vi "Solartron 1260 freq scan.vi"(0 "VISA resource name":refnum<visa-resource-name>, 11 "error in (no error)":errorcluster) -> ()   [LabVIEW 2014]
doc: "This VI configures and reads back a single measurement. \n\nNote:\nYou might need to extend the timeout set in the Wait Conditions subVI."
uses:
  <vilib>/Utility/file.llb/Write To Spreadsheet File (string).vi
  <instrlib>/Solartron 1260/Solartron 1260.lvlib
panel:
  out "scan time (hrs)":dbl
  out "scan time (min)":dbl
  in  "stop":bool
  out "resonant freq (Hz)":dbl format="%#_13f"
  out "Step size (Hz)":dbl
  out "XY Graph 3":cluster{dbl[], dbl[]}[](graph)
  in  "Frequency options":T1 {"Start freq (Hz)" format="%#_8f"; "End freq (Hz)" format="%#_8f"}
  in  "Cluster":cluster{"DC Bias (V)":dbl, "Amplitude (V)":dbl}={"DC Bias (V)"=0.0, "Amplitude (V)"=1.0} {"Amplitude (V)" min=0.0 max=3.0 format="%^.3e"; "DC Bias (V)" min=-42.0 max=42.0 format="%^.3e"}
  in  "Variable, result source, citcuit":T2
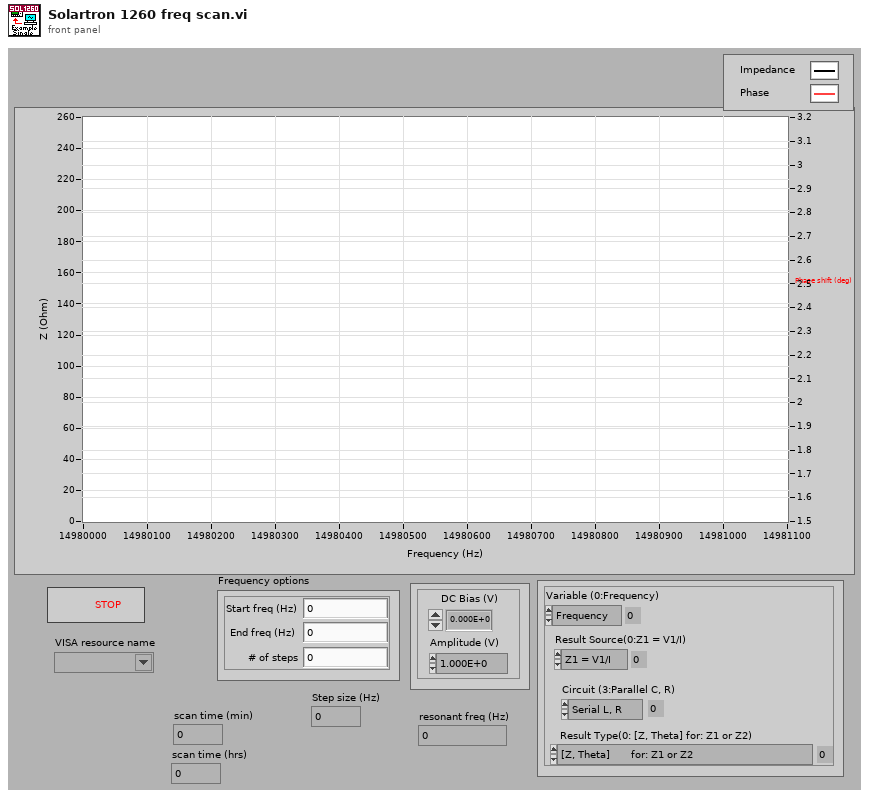
[diagram p1: front panel]
types:
  T1 = cluster{"End freq (Hz)":dbl, "Start freq (Hz)":dbl, "# of steps":dbl}
  T2 = cluster{"Variable (0:Frequency)":enum16{"Frequency", "Amplitude", "Baise"}, "Result Source(0:Z1 = V1/I)":enum16{"Z1 = V1/I", "Y1 = I/V1", "Z2 = V2/I", "Y2 = I/V2", "Function (  )", "V1", "V2", "V1/V2", "V2/V1", " I"}, "Circuit (3:Parallel C, R)":enum16{"Serial L, R", "Serial C, R", "Parallel L, R", "Parallel C, R", "Auto"}, "Result Type(0: [Z, Theta] for: Z1 or Z2)":enum16{"[Z, Theta]       for: Z1 or Z2", "[Y, Theta]       for: Y1 or Y2", "[r, Theta]        for: Fnc( ), V1, V2, V1/V2, V2/V1 or I", "[r(dB), Theta]  for: Fnc( ), V1, V2, V1/V2 or V2/V1", "[r, t]                 for: Fnc( ), V1, V2, V1/V2 or V2/V1", "[r (dB), t]          for: Fnc( ), V1, V2, V1/V2 or V2/V1", "[L(or C), R]      for: Z1, Y1, Z2, Y2 or Fnc( )", "[L(or C), Q]      for: Z1, Y1, Z2, Y2 or Fnc( )", "[L(or C), D]      for: Z1, Y1, Z2, Y2 or Fnc( ) ", "[R, X]              for: Z1 or Z2", "[G, B]              for: Y1 or Y2", "[a, b]               for: Fnc( ), V1, V2, V1/V2, V2/V1 or I"}}
  T3 = enum16{"Off", "All", "Fail", "Pass", "Dump", "Dump all", "Plotter"}
  T4 = enum16{"Z1 = V1/I", "Y1 = I/V1", "Z2 = V2/I", "Y2 = I/V2", "Function (  )", "V1", "V2", "V1/V2", "V2/V1", " I"}
  T5 = enum16{"Serial L, R", "Serial C, R", "Parallel L, R", "Parallel C, R", "Auto"}
  T6 = enum16{"[Z, Theta]       for: Z1 or Z2", "[Y, Theta]       for: Y1 or Y2", "[r, Theta]        for: Fnc( ), V1, V2, V1/V2, V2/V1 or I", "[r(dB), Theta]  for: Fnc( ), V1, V2, V1/V2 or V2/V1", "[r, t]                 for: Fnc( ), V1, V2, V1/V2 or V2/V1", "[r (dB), t]          for: Fnc( ), V1, V2, V1/V2 or V2/V1", "[L(or C), R]      for: Z1, Y1, Z2, Y2 or Fnc( )", "[L(or C), Q]      for: Z1, Y1, Z2, Y2 or Fnc( )", "[L(or C), D]      for: Z1, Y1, Z2, Y2 or Fnc( ) ", "[R, X]              for: Z1 or Z2", "[G, B]              for: Y1 or Y2", "[a, b]               for: Fnc( ), V1, V2, V1/V2, V2/V1 or I"}
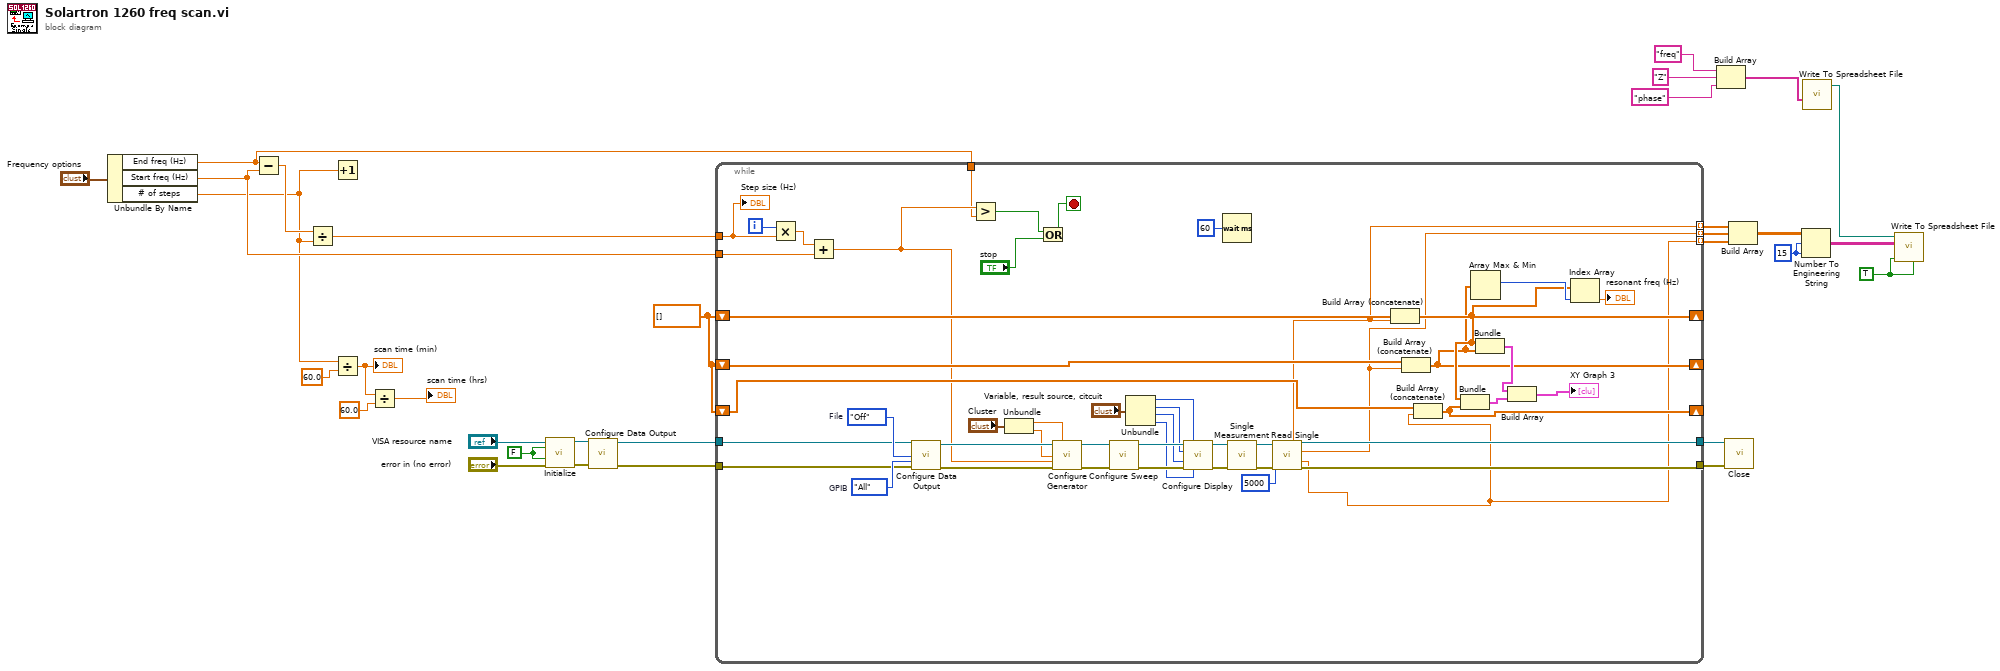
[diagram p0: block diagram]
diagram:
  w6 = TRUE ("append to file? (new file:F)")
  w14 = i16 15 ("precision (6)")
  w19 = dbl[] []
  w29 = FALSE ("ID Query (T: Check)")
  n1 = Unbundle By Name("Frequency options") -> ("End freq (Hz)"=w7:dbl, "Start freq (Hz)"=w21:dbl, "# of steps"=w4:dbl)
  n2 = Subtract(x=w7, y=w21) -> (x-y=w32:dbl)
  n3 = Divide(x=w32, y=w4) -> (x/y=w20:dbl)
  n4 = Increment(x=w4) -> ()  [unwired: 1 out]
  n5 = Divide(x=w4, y=60.0) -> (x/y=w2:dbl)
  "scan time (min)" <- w2
  n6 = Divide(x=w2, y=60.0) -> (x/y=→"scan time (hrs)":dbl)
  n7 = call <instrlib>:"Initialize.vi"("VISA resource name"="VISA resource name", "ID Query (T: Check)"=w29, "Reset (T: Reset)"=w29, "error in (no error)"="error in (no error)") -> ("VISA resource name out"=w25:refnum<visa-resource-name>, "error out"=w26:errorcluster)  [unwired: 10 in]
  n8 = call <instrlib>:"Configure Data Output.vi"("VISA resource name"=w25, "error in (no error)"=w26) -> ("VISA resource name out"=w24:refnum<visa-resource-name>, "error out"=w23:errorcluster)  [unwired: 12 in]
  n9 = while {
    tunnel: [w62] -> w31
    tunnel: [w61] -> w30
    tunnel: w24 -> [w64]
    tunnel: w23 -> [w63]
    tunnel: w21 -> [w78]
    shift-right: [w43] -> _
    shift-left: w19 -> [w60]
    shift-right: [w41] -> _
    shift-left: w19 -> [w59]
    tunnel: w20 -> [w50]
    shift-right: [w46] -> _
    shift-left: w19 -> [w47]
    tunnel: [w40] -> w18 mode=indexing
    tunnel: [w34] -> w17 mode=indexing
    tunnel: [w33] -> w16 mode=indexing
    tunnel: w7 -> [w36]
    i -> [w80]
    stop <- w39 stop-if-true
    w66 = T3."All"  # GPIB
    w67 = enum16{"Off", "All", "Fail", "Pass"}."Off"  # File
    n10 = Multiply(x=w80, y=w50) -> (x*y=w79:dbl)
    n11 = Add(x=w79, y=w78) -> (x+y=w37:dbl)
    n12 = call <instrlib>:"Configure Data Output.vi"("VISA resource name"=w64, "File (1:All)"=w67, "GPIB (1:All)"=w66, "error in (no error)"=w63) -> ("VISA resource name out"=w76:refnum<visa-resource-name>, "error out"=w77:errorcluster)  [unwired: 10 in]
    n13 = Greater?(x=w37, y=w36) -> (0:w35:bool)
    n14 = Unbundle("Cluster") -> ("DC Bias (V)"=w53:dbl, "Amplitude (V)"=w52:dbl)
    n15 = Or(x=w35, y="stop") -> (x .or. y?=w39:bool)
    n16 = call <instrlib>:"Configure Generator.vi"("VISA resource name"=w76, "Voltage Bias(0.0 V)"=w53, "Voltage Amplitude(1.0 V)"=w52, "Frequency(1.0 Hz)"=w37, "error in (no error)"=w77) -> ("VISA resource name out"=w75:refnum<visa-resource-name>, "error out"=w74:errorcluster)  [unwired: 9 in]
    n17 = call <instrlib>:"Configure Sweep.vi"("VISA resource name"=w75, "error in (no error)"=w74) -> ("VISA resource name out"=w72:refnum<visa-resource-name>, "error out"=w73:errorcluster)  [unwired: 12 in]
    n18 = Unbundle("Variable, result source, citcuit") -> ("Variable (0:Frequency)"=w57:enum16{"Frequency", "Amplitude", "Baise"}, "Result Source(0:Z1 = V1/I)"=w55:T4, "Circuit (3:Parallel C, R)"=w56:T5, "Result Type(0: [Z, Theta] for: Z1 or Z2)"=w51:T6)
    n19 = call <instrlib>:"Configure Display.vi"("VISA resource name"=w72, "Variable (0:Frequency)"=w57, "Result Source(0:Z1 = V1/I)"=w55, "Circuit (3:Parallel C, R)"=w56, "error in (no error)"=w73, "Result Type(0: [Z, Theta] for: Z1 or Z2)"=w51) -> ("VISA resource name out"=w71:refnum<visa-resource-name>, "error out"=w70:errorcluster)  [unwired: 8 in]
    n20 = Wait (ms)(milliseconds to wait=u32 60) -> ()  [unwired: 1 out]
    n21 = call <instrlib>:"Single Measurement.vi"("VISA resource name"=w71, "error in (no error)"=w70) -> ("VISA resource name out"=w68:refnum<visa-resource-name>, "error out"=w69:errorcluster)  [unwired: 12 in]
    n22 = call <instrlib>:"Read Single.vi"("VISA resource name"=w68, "timeout ms (5000)"=u32 5000, "error in (no error)"=w69) -> ("Variable"=w40:dbl, "VISA resource name out"=w61:refnum<visa-resource-name>, "Parameter 1"=w34:dbl, "Parameter2"=w33:dbl, "error out"=w62:errorcluster)  [unwired: 6 in, 2 out]
    n23 = Build Array (concatenate)(w60, w40) -> (w43:dbl[])
    n24 = Build Array (concatenate)(w59, w34) -> (w41:dbl[])
    n25 = Build Array (concatenate)(w47, w33) -> (w46:dbl[])
    n26 = Bundle(w43, w46) -> (w48:cluster{dbl[], dbl[]})  [unwired: 1 in]
    n27 = Array Max & Min(array=w41) -> (max index (indices)=w44:i32)  [unwired: 3 out]
    n28 = Bundle(w43, w41) -> (w49:cluster{dbl[], dbl[]})  [unwired: 1 in]
    n29 = Build Array(w49, w48) -> (→"XY Graph 3":cluster{dbl[], dbl[]}[])
    n30 = Index Array(array=w43, index=w44) -> (element=→"resonant freq (Hz)":dbl)
    "Step size (Hz)" <- w50
  }
  n31 = Build Array("freq", "Z", "phase") -> (w11:string[])
  n32 = call <instrlib>:"Close.vi"("VISA resource name"=w30, "error in (no error)"=w31) -> ()  [unwired: 13 in, 1 out]
  n33 = Build Array(w18, w17, w16) -> (w15:dbl[][])
  n34 = Number To Engineering String(2:w14, 3:w14, 4:w15) -> (0:w13:string[][])  [unwired: 1 in]
  n35 = call-poly <vilib>:"Write To Spreadsheet File.vi"("1D data"=w11) -> ("new file path (Not A Path if cancelled)"=w12:path)  [unwired: 7 in]
  n36 = call-poly <vilib>:"Write To Spreadsheet File.vi"("transpose? (no:F)"=w6, "append to file? (new file:F)"=w6, "2D data"=w13, "file path (dialog if empty)"=w12) -> ()  [unwired: 4 in, 1 out]
